vi "Compile Status FIFO Indices.vi"(8 "error in (no error)":errorcluster, 11 "Device Item Ref in":T2 format="%.0x") -> (0 "error out":errorcluster, 2 "FIFO Indices":T1, 3 "Device Item Ref out":T2 format="%.0x")   [LabVIEW 2017, in "SLSC Switch System Explorer.lvlib"]
uses:
  SLSC Switch System Explorer.lvlib
  <vilib>/NI Veristand/Custom Device API/Custom Device Item Ref.ctl
  Shared/FIFO Indices.ctl
  Scripting/SLSC Scripting Constants.vi
  <vilib>/NI Veristand/Custom Device Tools/Custom Device Utility Library/Custom Device Utility Library.lvlib
  <vilib>/NI Veristand/Custom Device API/Custom Device API.lvlib
  Scripting/SLSC Switch Scripting.lvlib
  Shared/SLSC Switch Shared.lvlib
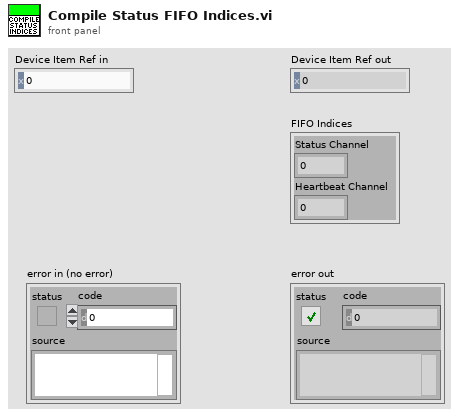
[diagram p1: front panel]
types:
  T1 = typedef "SLSC Switch Shared.lvlib/FIFO Indices.ctl" = cluster{"Status Channel":i32, "Heartbeat Channel":i32}
  T2 = typedef "Custom Device API.lvlib/Custom Device Item Ref.ctl" = u64
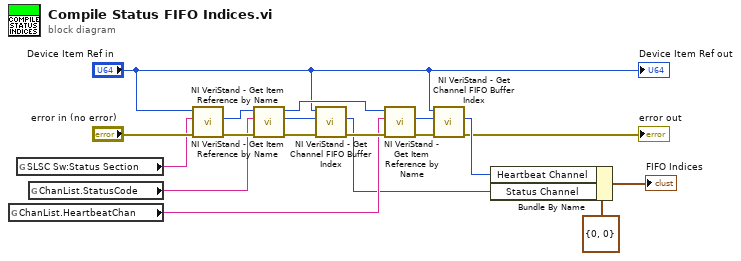
[diagram p0: block diagram]
diagram:
  n1 = global read "SLSC Scripting Constants.vi" "ChanList.HeartbeatChan"() -> (w9:string)
  n2 = global read "SLSC Scripting Constants.vi" "SLSC Sw:Status Section"() -> (w17:string)
  n3 = global read "SLSC Scripting Constants.vi" "ChanList.StatusCode"() -> (w14:string)
  n4 = call <vilib>:"NI VeriStand - Get Item Reference by Name.vi"("error in (no error)"="error in (no error)", "Item Name"=w17, "Parent Ref in"="Device Item Ref in") -> ("error out"=w16:errorcluster, "Item Ref"=w15:T2)  [unwired: 5 in, 2 out]
  n5 = call <vilib>:"NI VeriStand - Get Item Reference by Name.vi"("error in (no error)"=w16, "Item Name"=w14, "Parent Ref in"=w15) -> ("error out"=w13:errorcluster, "Item Ref"=w12:T2, "Parent Ref out"=w10:T2)  [unwired: 5 in, 1 out]
  n6 = call <vilib>:"NI VeriStand - Get Channel FIFO Buffer Index.vi"("error in"=w13, "Channel Ref"=w12, "Device Ref in"="Device Item Ref in") -> ("error out"=w11:errorcluster, "Channel FIFO Buffer Index"=w4:i32)  [unwired: 4 in, 3 out]
  n7 = call <vilib>:"NI VeriStand - Get Item Reference by Name.vi"("error in (no error)"=w11, "Item Name"=w9, "Parent Ref in"=w10) -> ("error out"=w8:errorcluster, "Item Ref"=w7:T2)  [unwired: 5 in, 2 out]
  n8 = call <vilib>:"NI VeriStand - Get Channel FIFO Buffer Index.vi"("error in"=w8, "Channel Ref"=w7, "Device Ref in"="Device Item Ref in") -> ("error out"=→"error out":errorcluster, "Channel FIFO Buffer Index"=w5:i32)  [unwired: 4 in, 3 out]
  n9 = Bundle By Name(cluster=T1 {"Status Channel"=0, "Heartbeat Channel"=0} ("FIFO Indices"), "Heartbeat Channel"=w5, "Status Channel"=w4) -> (→"FIFO Indices":T1)
  "Device Item Ref out" <- "Device Item Ref in"
